vi "snap_single_image.vi"(8 "error in (no error)":errorcluster, 11 "Session In":T1) -> (0 "error out":errorcluster, 3 "Image Out":T2)   [LabVIEW 2019]
uses:
  <vilib>/vision/Image Controls.llb/IMAQ Image.ctl
  <vilib>/userdefined/High Color/IMAQdx.ctl
  <vilib>/vision/driver/IMAQdx.llb/IMAQdx Acquisition Mode.ctl
  <vilib>/vision/driver/NI_Vision_Acquisition_Software.lvlib
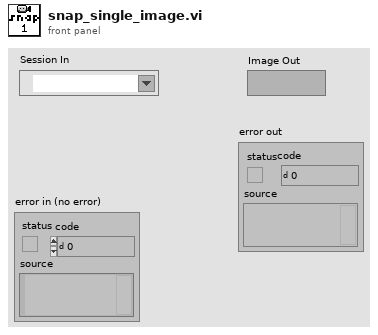
[diagram p1: front panel]
types:
  T1 = typedef "IMAQdx.ctl" = refnum<k21>
  T2 = typedef "IMAQ Image.ctl" = refnum<image>
  T3 = typedef "Image Type" = u32
  T4 = typedef "NI_Vision_Acquisition_Software.lvlib/IMAQdx Acquisition Mode.ctl" = enum32{"One Shot", "Continuous"}
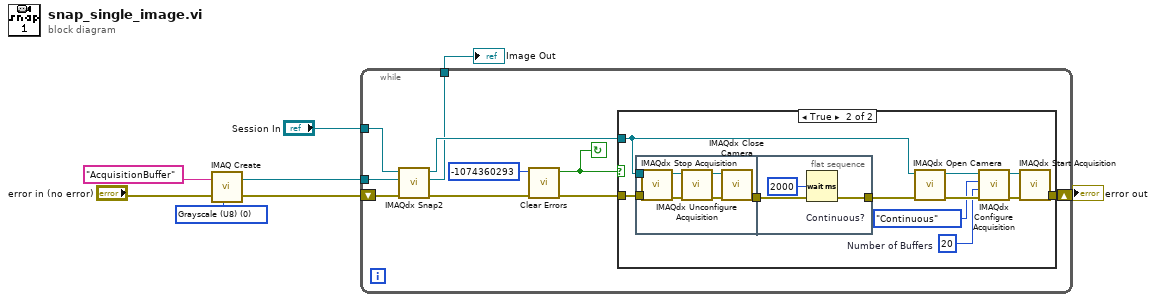
[diagram p0: block diagram]
diagram:
  w7 = T3 0 items=["Grayscale (U8)", "Grayscale (I16)", "Grayscale (SGL)", "Complex (CSG)", "RGB (U32)", "HSL (U32)", "RGB (U64)"] ("Image Type")
  n1 = call "IMAQ Create"("Image Name"="AcquisitionBuffer", "Image Type"=w7, "error in (no error)"="error in (no error)") -> ("New Image"=w5:T2, "error out"=w3:errorcluster)  [unwired: 2 in]
  n2 = while {
    tunnel: "Session In" -> [w18]
    tunnel: w5 -> [w17]
    shift-right: [w11] -> w2
    shift-left: w3 -> [w16]
    tunnel: [w9] -> w1
    stop <- w13 continue-if-true
    n3 = call <vilib>:"IMAQdx Snap2.vi"("error in"=w16, "Image In"=w17, "Session In"=w18) -> ("error out"=w15:errorcluster, "Image Out"=w9:T2, "Session Out"=w10:T1)  [unwired: 6 in]
    n4 = call <vilib>:"Clear Errors.vi"("error in (no error)"=w15, "specific error code to clear (0: all)"=-1074360293) -> ("error out"=w12:errorcluster, "specific error cleared?"=w13:bool)  [unwired: 4 in]
    n5 = case shown="True" w13 {
      tunnel: w12 -> [w19 w24]
      tunnel: [w19 w22] -> w11
      tunnel: w10 -> [_ w21]
      frame False {
      }
      frame True {
        w26 = u32 20  # Number of Buffers
        w25 = IMAQdx_Acquisition_Mode."Continuous"  # Continuous?
        n6 = flat-sequence {
          tunnel: w24 -> [w33]
          tunnel: w21 -> [w31]
          tunnel: [w32] -> w20
          tunnel: [w39] -> w23
          tunnel: w20 -> [w39]
          frame #0 {
            n7 = call <vilib>:"IMAQdx Stop Acquisition.vi"("error in"=w33, "Session In"=w31) -> ("error out"=w34:errorcluster, "Session Out"=w35:T1)  [unwired: 8 in]
            n8 = call <vilib>:"IMAQdx Unconfigure Acquisition.vi"("error in"=w34, "Session In"=w35) -> ("error out"=w37:errorcluster, "Session Out"=w36:T1)  [unwired: 8 in]
            n9 = call <vilib>:"IMAQdx Close Camera.vi"("error in"=w37, "Session In"=w36) -> ("error out"=w32:errorcluster)  [unwired: 9 in]
          }
          frame #1 {
            n10 = Wait (ms)(milliseconds to wait=u32 2000) -> ()  [unwired: 1 out]
          }
        }
        n11 = call <vilib>:"IMAQdx Open Camera.vi"("error in"=w23, "Session In"=w21) -> ("error out"=w28:errorcluster, "Session Out"=w27:T1)  [unwired: 8 in]
        n12 = call <vilib>:"IMAQdx Configure Acquisition.vi"("error in"=w28, "Number of Buffers"=w26, "Continuous?"=w25, "Session In"=w27) -> ("error out"=w29:errorcluster, "Session Out"=w30:T1)  [unwired: 6 in]
        n13 = call <vilib>:"IMAQdx Start Acquisition.vi"("error in"=w29, "Session In"=w30) -> ("error out"=w22:errorcluster)  [unwired: 8 in, 1 out]
      }
    }
  }
  "error out" <- w2
  "Image Out" <- w1
